vi "AKIP_initialize.vi"(8 "error in (no error)":errorcluster, 11 "VISA Refnum in":refnum<visa-resource-name>="AKIP") -> (0 "error out":errorcluster, 3 "VISA Refnum out":refnum<visa-resource-name>="AKIP")   [LabVIEW 2017]
uses:
  <vilib>/Instr/_visa.llb/VISA Open Access Mode.ctl
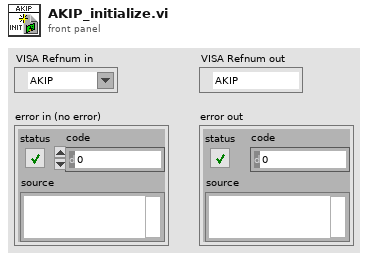
[diagram p1: front panel]
types:
  T1 = typedef "VISA Open Access Mode.ctl" = u32
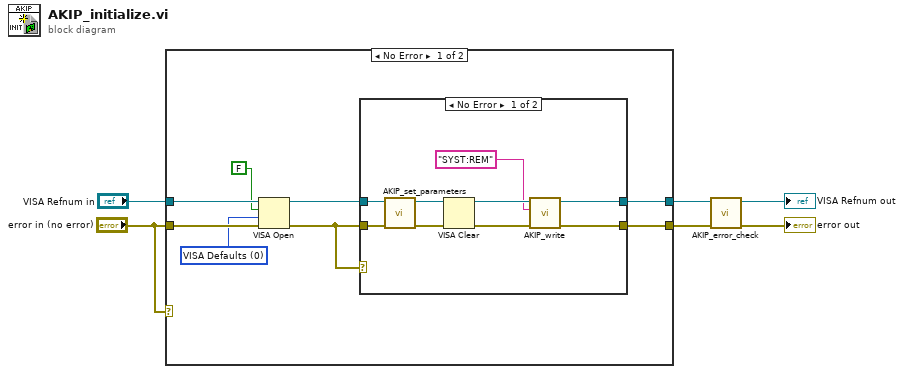
[diagram p0: block diagram]
diagram:
  n1 = case shown="No Error" "error in (no error)" {
    tunnel: [w14 w26] -> w3
    tunnel: [w13 w27] -> w4
    tunnel: "error in (no error)" -> [w11 w26]
    tunnel: "VISA Refnum in" -> [w10 w27]
    frame No Error {
      w9 = T1 0 items=["VISA Defaults"=0, "Exclusive Lock"=1, "Load Configured Settings"=4] ("Access Mode")
      n2 = VISA Open(duplicate session (F)=FALSE, access mode=w9, error in (no error)=w11, VISA resource name=w10) -> (VISA resource name=w12:refnum<visa-resource-name>, error out=w7:errorcluster)  [unwired: 1 in]
      n3 = case shown="No Error" w7 {
        tunnel: [w16 w24] -> w14
        tunnel: [w17 w25] -> w13
        tunnel: w7 -> [w23 w24]
        tunnel: w12 -> [w22 w25]
        frame No Error {
          n4 = call "AKIP_set_parameters.vi"("error in (no error)"=w23, "VISA Refnum in"=w22) -> ("error out"=w20:errorcluster, "VISA Refnum out"=w21:refnum<visa-resource-name>)  [unwired: 8 in]
          n5 = VISA Clear(VISA resource name=w21, error in (no error)=w20) -> (VISA resource name out=w18:refnum<visa-resource-name>, error out=w19:errorcluster)
          n6 = call "AKIP_write.vi"("error in (no error)"=w19, "write buffer"="SYST:REM", "VISA Refnum in"=w18) -> ("error out"=w16:errorcluster, "VISA Refnum out"=w17:refnum<visa-resource-name>)  [unwired: 7 in]
        }
        frame Error {
        }
      }
    }
    frame Error {
    }
  }
  n7 = call "AKIP_error_check.vi"("error in (no error)"=w3, "VISA Refnum in"=w4) -> ("error out"=→"error out":errorcluster, "VISA Refnum out"=→"VISA Refnum out":refnum<visa-resource-name>)  [unwired: 8 in]
